vi "Make Child Window.vi"(4 "error in (no error)":errorcluster, 6 "Name of Child Panel":string, 7 "Name of Parent Panel":string) -> (0 "error out":errorcluster)   [LabVIEW 2018]
doc: "Developer: Wayne Lootsma\nDate: 01/08/2003\nDescription:\nVi from NIs website for making an IMAQ window a child window, works only on Windows systems. Here is the original text:\nIMAQ MakeChild will allow you to embed your IMAQ Vision display into any vi's Front Panel.\n\nIt is okay to use IMAQ WindMove, IMAQ WindSize, IMAQ WindSetup, etc to define properties of the child window before calling this function. Doing so will allow you to customize the look and feel of your user interface.\n\nParent Panel Name is the name of the vi into which the IMAQ Vision window is to be embedded. This vi must be loaded into memory. \n\nWindow Number is the IMAQ Vision window number of the window which is to be made a child. This number is specified in IMAQ Create. \n\n\nDialog Panel: False\nGUI Panel: False\n\nDLL Description:\nInterface with a window for an IMAQ window.\n\nParty's Responsible: Microsoft Corp.\nDLL Filename: User32.dll\nDLL Location: C:\\Windows\\System\nProduct Name, Compiler and Version Number: Microsoft Visual C++, C Compiler V 2.0\nOperating System: Windows NT, 2000.\nLast Date Modified: 03/26/2003"
uses:
  User32.dll
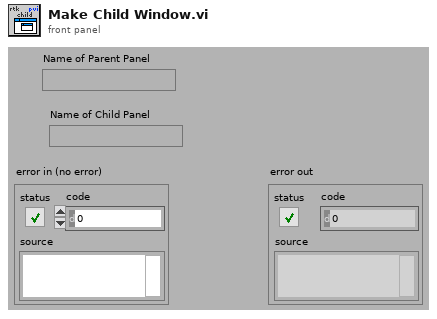
[diagram p1: front panel]
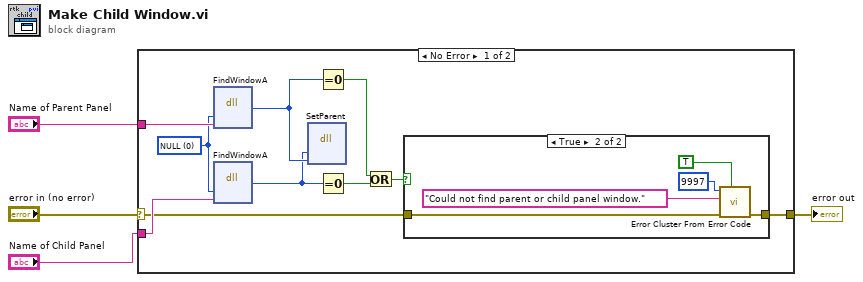
[diagram p0: block diagram]
diagram:
  n1 = case shown="No Error" "error in (no error)" {
    selector: "error in (no error)" -> [w10 w21]
    tunnel: [w8 w21] -> w4
    tunnel: "Name of Parent Panel" -> [w13 _]
    tunnel: "Name of Child Panel" -> [w11 _]
    frame No Error {
      w12 = 0 items=["NULL"]
      n2 = dll-call lib="user32.dll" fn="FindWindowA" label="FindWindow"("lpszClassName"=w12, "lpszWindowName"=w13) -> ("hWnd"=w14:u32)  [unwired: 5 in, 2 out]
      n3 = dll-call lib="User32.dll" fn="FindWindowA" label="FindWindow"("lpszClassName"=w12, "lpszWindowName"=w11) -> ("hWnd"=w9:u32)  [unwired: 5 in, 2 out]
      n4 = dll-call lib="user32.dll" fn="SetParent"("Child"=w9, "NewParent"=w14) -> ()  [unwired: 6 in, 2 out]
      n5 = Equal To 0?(x=w14) -> (x = 0?=w7:bool)
      n6 = Equal To 0?(x=w9) -> (x = 0?=w6:bool)
      n7 = Or(x=w7, y=w6) -> (x .or. y?=w5:bool)
      n8 = case shown="True" w5 {
        tunnel: w10 -> [w15 w18]
        tunnel: [w15 w16] -> w8
        frame False {
        }
        frame True {
          n9 = call <vilib>:"Error Cluster From Error Code.vi"("show call chain? (False)"=TRUE, "error in (no error)"=w18, "error message (\"\")"="Could not find parent or child panel window." ("error message (\"\")"), "error code (0)"=9997) -> ("error out"=w16:errorcluster)  [unwired: 5 in]
        }
      }
    }
    frame Error {
    }
  }
  "error out" <- w4
